vi "write_markerdata.vi"(0 "Data to save in":dbl[][](array[numeric]), 1 "Connected to Unity last call? In":bool, 2 "Connected to Unity via TCP?":bool, 3 "Host folder":path=path "C:/Users/User/Documents/GitHub/RobUST/Labview/RobUST_3D/Recorded Data", 4 "Unity task info string":string, 5 "DesiredTensions":dbl[](array[numeric]), 6 "Current save file in":path, 7 "CurrentTensions":dbl[](array[numeric]), 8 "New task info string flag in":bool, 9 "Last Vicon frame read":u32, 10 "Task has ended flag":bool) -> (14 "Connected to Unity last call? Out":bool, 15 "Current save file out":path, 16 "Data to save":dbl[][](array[numeric]), 17 "New task info string flag out":bool, 18 "Task had ended flag out":bool)   [LabVIEW 2024]
panel:
  in  "Actively record tensions":bool
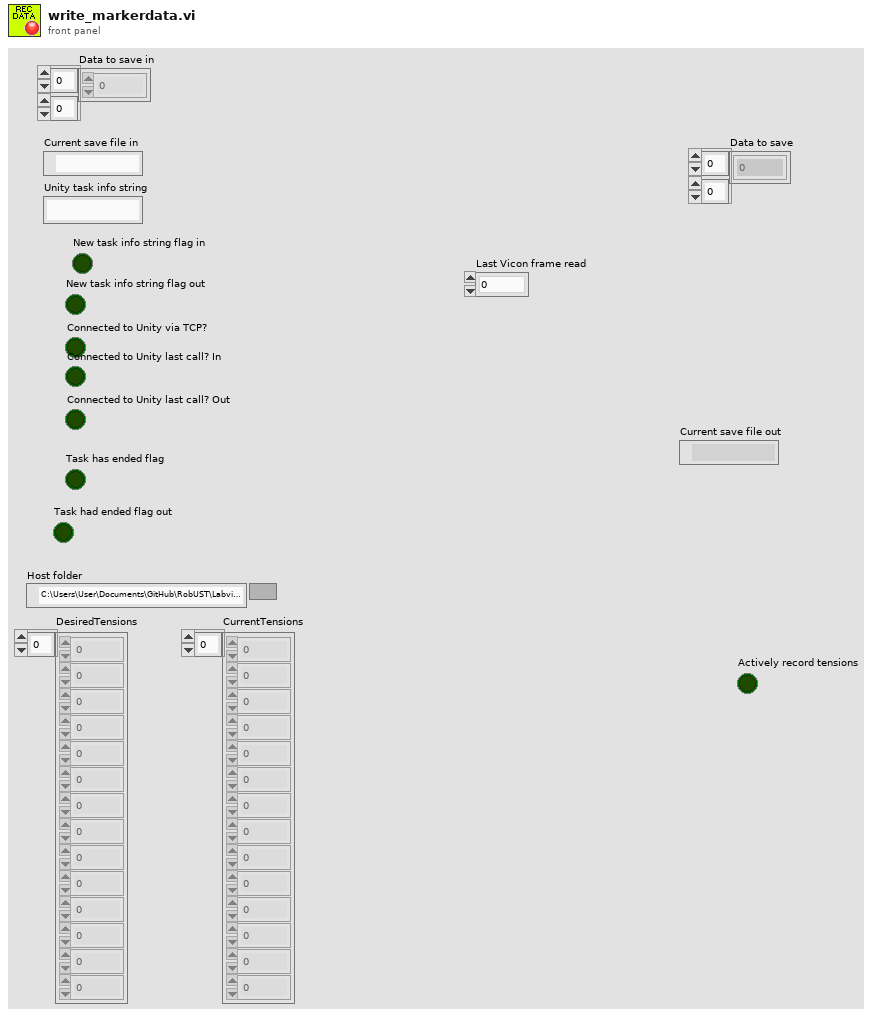
[diagram p1: front panel]
types:
  T1 = enum16{"open", "replace", "create", "open or create", "replace or create", "replace or create with confirmation"}
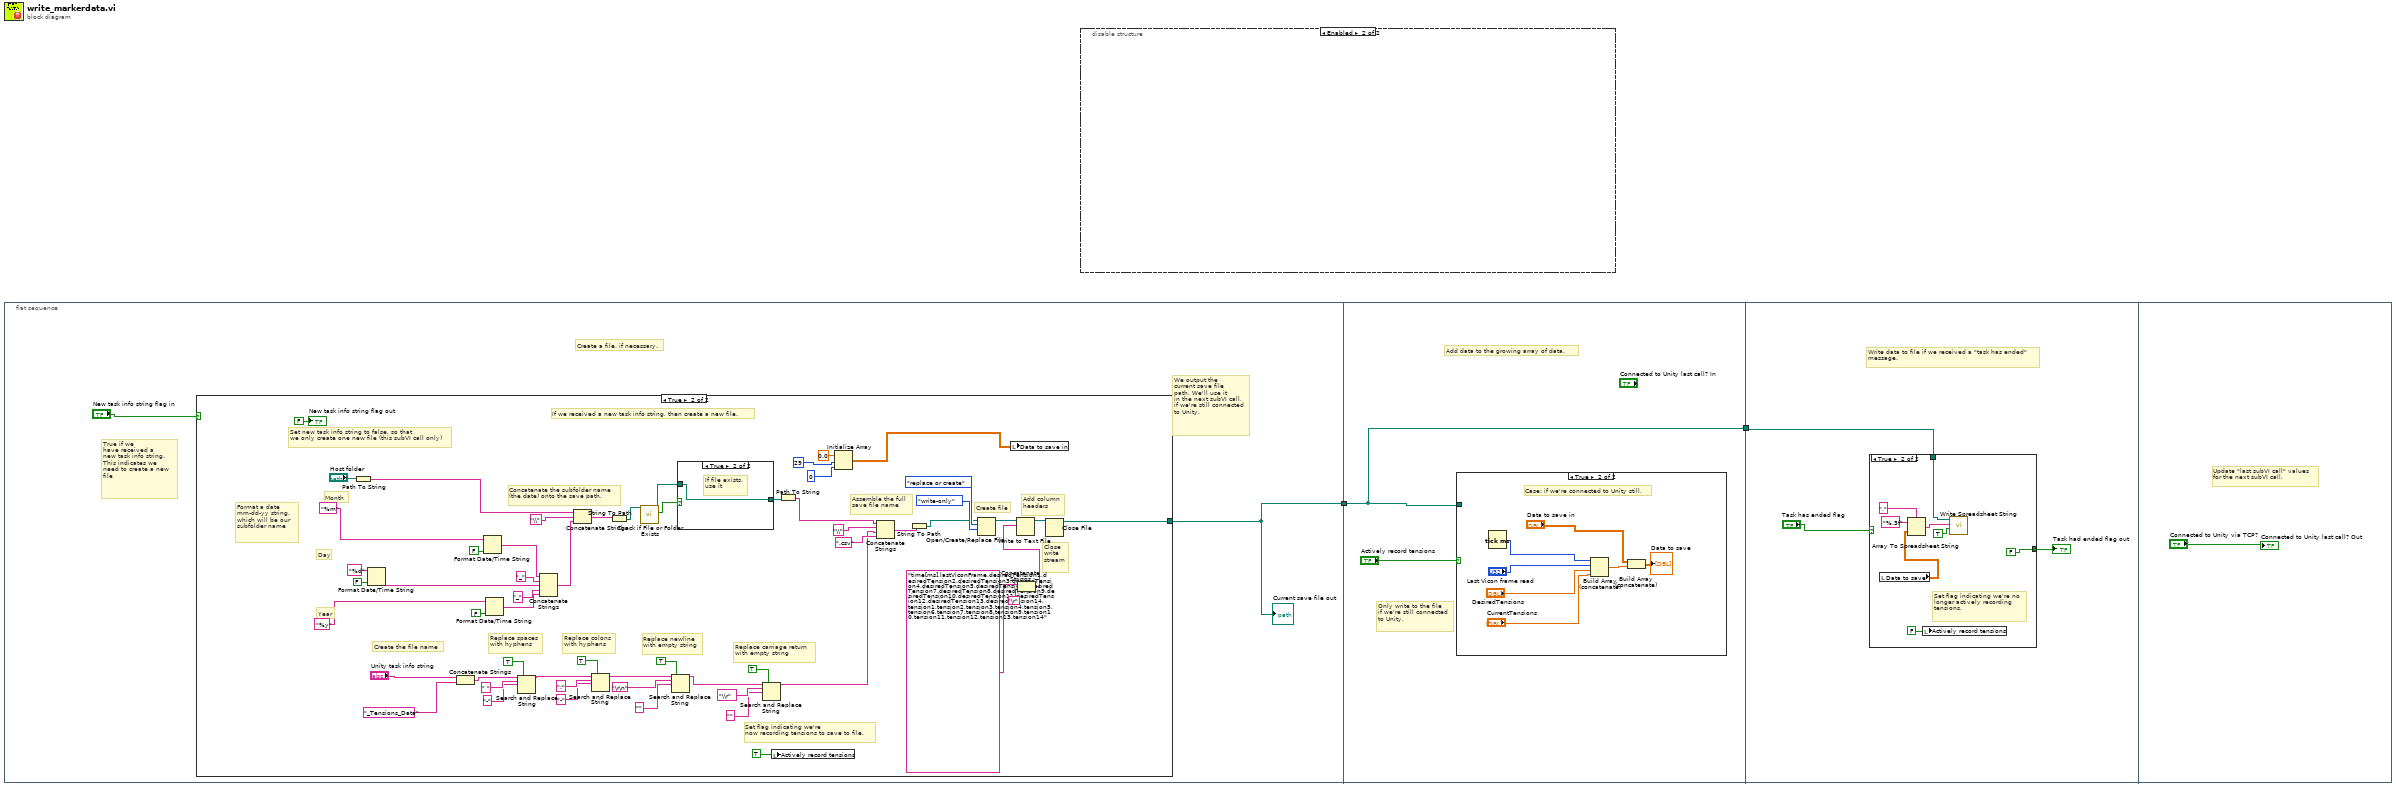
[diagram p0: block diagram]
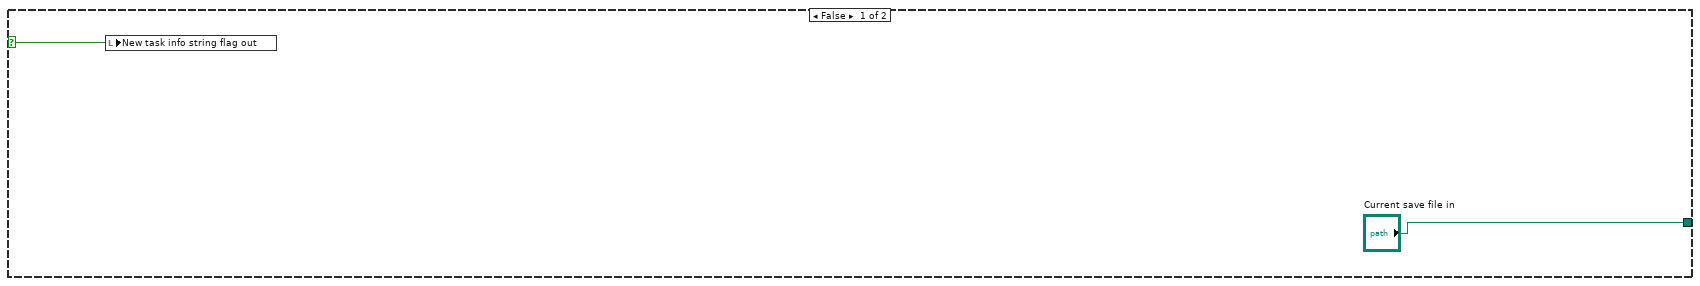
[diagram p2: hidden frame]
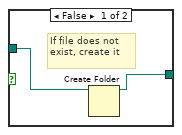
[diagram p3: hidden frame]
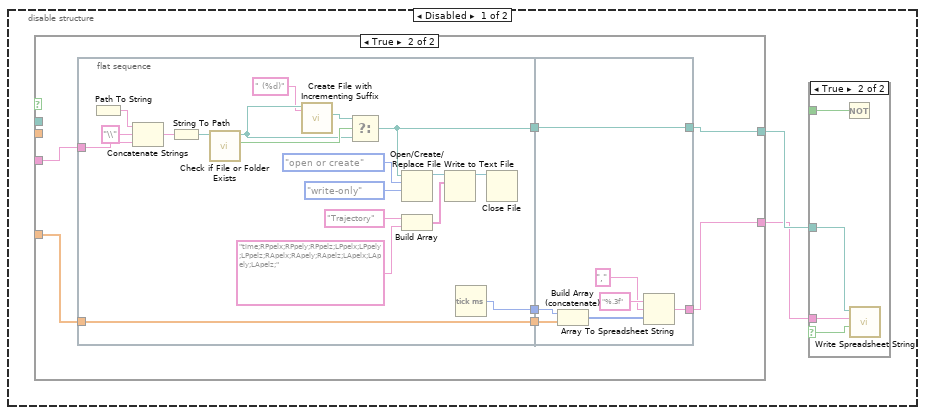
[diagram p6: hidden frame]
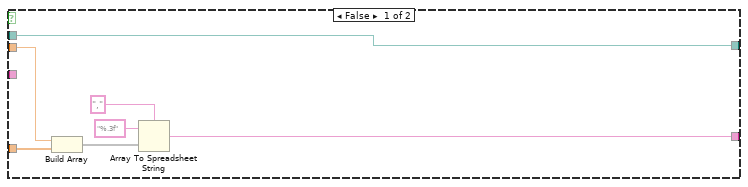
[diagram p7: hidden frame]
diagram:
  n1 = flat-sequence {
    tunnel: [w4] -> w2
    tunnel: w2 -> [w69]
    tunnel: [w69] -> w1
    tunnel: w1 -> [w79]
    frame #0 {
      # "We output the \ncurrent save file\npath. We'll use it \nin the next subVI call,\nif we're still connected\nto Unity."
      # "True if we \nhave received a \nnew task info string. \nThis indicates we \nneed to create a new \nfile"
      # "Create a file, if necessary."
      n2 = case shown="True" "New task info string flag in" {
        selector: "New task info string flag in" -> [w5 _]
        tunnel: ["Current save file in" w41] -> w4
        frame False {
          n3 = local write "New task info string flag out"(w5) -> ()
        }
        frame True {
          # "Day"
          # "Replace carriage return\nwith empty string"
          # "Replace newline\nwith empty string"
          # "Set flag indicating we're \nnow recording tensions to save to file."
          # "Set new task info string to false, so that\nwe only create one new file (this subVI call only)"
          # "Replace colons\nwith hyphens"
          # "Replace spaces\nwith hyphens"
          # "Close \nwrite\nstream"
          # "Add column\nheaders"
          # "Create file"
          # "Assemble the full \nsave file name"
          # "Create the file name"
          # "If we received a new task info string, then create a new file."
          # "Concatenate the subfolder name\n(the date) onto the save path."
          # "Format a date\nmm-dd-yy string, \nwhich will be our \nsubfolder name"
          # "Year"
          # "Month"
          n4 = Path To String(path="Host folder") -> (string=w63:string)
          n5 = Format Date/Time String(time format string (%c)="%d", UTC format=FALSE) -> (date/time string=w8:string)  [unwired: 1 in]
          n6 = Concatenate Strings("Unity task info string", "_Tensions_Data" ("string")) -> (w40:string)
          n7 = Format Date/Time String(time format string (%c)="%m", UTC format=FALSE) -> (date/time string=w62:string)  [unwired: 1 in]
          n8 = Format Date/Time String(time format string (%c)="%y", UTC format=FALSE) -> (date/time string=w9:string)  [unwired: 1 in]
          n9 = Search and Replace String(replace all?=TRUE ("replace all? (F)"), input string=w40, search string=" ", replace string="-" ("replace string (\"\")")) -> (result string=w33:string)  [unwired: 4 in, 3 out]
          n10 = Concatenate Strings(w62, "_" ("string"), w8, "_" ("string"), w9) -> (w64:string)
          n11 = Concatenate Strings(w63, "\\" ("string"), w64) -> (w49:string)
          n12 = Search and Replace String(replace all?=TRUE ("replace all? (F)"), input string=w33, search string=":", replace string="-" ("replace string (\"\")")) -> (result string=w18:string)  [unwired: 4 in, 3 out]
          n13 = String To Path(string=w49) -> (path=w52:path)
          n14 = call <vilib>:"Check if File or Folder Exists.vi"("path"=w52) -> ("file or folder exists?"=w51:bool, "dup path"=w50:path)  [unwired: 8 in, 1 out]
          n15 = Search and Replace String(replace all?=TRUE ("replace all? (F)"), input string=w18, search string="\r\n", replace string="" ("replace string (\"\")")) -> (result string=w14:string)  [unwired: 4 in, 3 out]
          n16 = case shown="True" w51 {
            tunnel: w50 -> [w66 w67]
            tunnel: [w65 w67] -> w48
            frame False {
              # "If file does not\nexist, create it"
              n17 = Create Folder(path (use dialog)=w66) -> (created path=w65:path)  [unwired: 2 in, 2 out]
            }
            frame True {
              # "If file exists, \nuse it"
            }
          }
          n18 = Search and Replace String(replace all?=TRUE ("replace all? (F)"), input string=w14, search string="\\r", replace string="" ("replace string (\"\")")) -> (result string=w13:string)  [unwired: 4 in, 3 out]
          n19 = local write "Actively record tensions"(TRUE ("Actively record tensions")) -> ()
          n20 = Path To String(path=w48) -> (string=w47:string)
          n21 = Initialize Array(0.0 ("element"), 29 ("dimension size"), 0 ("dimension size")) -> (w30:dbl[][])
          n22 = Concatenate Strings(w47, "\\" ("string"), w13, ".csv" ("string")) -> (w53:string)
          n23 = String To Path(string=w53) -> (path=w43:path)
          n24 = Open/Create/Replace File(file path (use dialog)=w43, operation (0:open)=T1."replace or create", access (0:read/write)=enum16{"read/write", "read-only", "write-only"}."write-only") -> (refnum out=w44:refnum<file>)  [unwired: 3 in, 2 out]
          n25 = local write "Data to save in"(w30) -> ()
          n26 = Concatenate Strings("time[ms],lastViconFrame,desiredTension1,desiredTension2,desiredTension3,desiredTension4,desiredTension5,desiredTension6,desiredTension7,desiredTension8,desiredTension9,desiredTension10,desiredTension11,desiredTension12,desiredTension13,desiredTension14, tension1,tension2,tension3,tension4,tension5,tension6,tension7,tension8,tension9,tension10,tension11,tension12,tension13,tension14" ("String"), "\r") -> (w27:string)
          n27 = Write to Text File(file (use dialog)=w44, text=w27) -> (refnum out=w42:refnum<file>)  [unwired: 2 in, 2 out]
          n28 = Close File(refnum=w42) -> (path=w41:path)  [unwired: 1 in, 1 out]
          "New task info string flag out" <- FALSE ("New task info string flag out")
        }
      }
      "Current save file out" <- w4
    }
    frame #1 {
      # "Add data to the growing array of data."
      # "Only write to the file\nif we're still connected\nto Unity."
      n29 = case shown="True" "Actively record tensions" {
        tunnel: w69 -> [_ _]
        frame False {
          # "If we're not currently connected \nto Unity, do nothing."
        }
        frame True {
          # "Case: if we're connected to Unity still."
          n30 = Tick Count (ms)() -> (millisecond timer value=w76:u32)
          n31 = Build Array (concatenate)(w76, "Last Vicon frame read", "DesiredTensions", "CurrentTensions") -> (w75:dbl[])
          n32 = Build Array (concatenate)("Data to save in", w75) -> (→"Data to save":dbl[][])
        }
      }
    }
    frame #2 {
      # "Write data to file if we received a \"task has ended\"\nmessage."
      n33 = case shown="True" "Task has ended flag" {
        selector: "Task has ended flag" -> [w80 _]
        tunnel: w79 -> [_ w84]
        tunnel: [w80 FALSE ("Task had ended flag out")] -> w77
        frame False {
        }
        frame True {
          # "Set flag indicating we're no\nlonger actively recording \ntensions."
          n34 = local read "Data to save"() -> (w83:dbl[][])
          n35 = Array To Spreadsheet String(delimiter (Tab)="," ("delimiter (\\t)"), array=w83, 3:"%.3f" ("format string")) -> (spreadsheet string=w88:string)
          n36 = local write "Actively record tensions"(FALSE ("Actively record tensions")) -> ()
          n37 = call <vilib>:"Write Spreadsheet String.vi"("append to file? (new file:F)"=TRUE, "spreadsheet string"=w88, "file path (dialog if empty)"=w84) -> ()  [unwired: 7 in, 2 out]
        }
      }
      "Task had ended flag out" <- w77
    }
    frame #3 {
      # "Update \"last subVI call\" values \nfor the next subVI call."
      "Connected to Unity last call? Out" <- "Connected to Unity via TCP?"
    }
  }
  n38 = disable-structure shown="Enabled" {
    frame Disabled {
      n39 = case shown="True" {
        selector: _ -> [_ _]
        tunnel: [w98 w104] -> w91
        tunnel: _ -> [w98 _]
        tunnel: _ -> [_ w105]
        tunnel: _ -> [w96 w100]
        tunnel: _ -> [w97 _]
        tunnel: [w94 w99] -> w90
        frame False {
          n40 = Build Array(w97, w96) -> (w95:void[])
          n41 = Array To Spreadsheet String(delimiter (Tab)="," ("delimiter (\\t)"), array=w95, 3:"%.3f" ("format string")) -> (spreadsheet string=w94:string)
        }
        frame True {
          n42 = flat-sequence {
            tunnel: w105 -> [w109]
            tunnel: [w113] -> w103
            tunnel: [w106] -> w102
            tunnel: [w111] -> w101
            tunnel: w100 -> [w111]
            tunnel: [w131] -> w104
            tunnel: w103 -> [w131]
            tunnel: w102 -> [w127]
            tunnel: w101 -> [w126]
            tunnel: [w125] -> w99
            frame #0 {
              n43 = Path To String() -> (string=w121:string)  [unwired: 1 in]
              n44 = Concatenate Strings(w121, "\\" ("string"), w109) -> (w120:string)
              n45 = String To Path(string=w120) -> (path=w123:path)
              n46 = call <vilib>:"Check if File or Folder Exists.vi"("path"=w123) -> ("file or folder exists?"=w124:bool, "dup path"=w119:path)  [unwired: 8 in, 1 out]
              n47 = call <vilib>:"Create File with Incrementing Suffix.vi"("format string (\" (%d)\")"=" (%d)" ("format string (\" (%d)\")"), "file path"=w119) -> ("actual path"=w118:path)  [unwired: 7 in, 2 out]
              n48 = Select(t=w118, s=w124, f=w119) -> (s? t:f=w113:path)
              n49 = Open/Create/Replace File(file path (use dialog)=w113, operation (0:open)=T1."open or create", access (0:read/write)=enum16{"read/write", "read-only", "write-only"}."write-only") -> (refnum out=w114:refnum<file>)  [unwired: 3 in, 2 out]
              n50 = Build Array("Trajectory" ("element"), "time;RPpelx;RPpely;RPpelz;LPpelx;LPpely;LPpelz;RApelx;RApely;RApelz;LApelx;LApely;LApelz;" ("String")) -> (w110:string[])
              n51 = Write to Text File(file (use dialog)=w114, text=w110) -> (refnum out=w112:refnum<file>)  [unwired: 2 in, 2 out]
              n52 = Tick Count (ms)() -> (millisecond timer value=w106:u32)
              n53 = Close File(refnum=w112) -> ()  [unwired: 1 in, 2 out]
            }
            frame #1 {
              n54 = Build Array (concatenate)(w127, w126) -> (w130:u32[])
              n55 = Array To Spreadsheet String(delimiter (Tab)="," ("delimiter (\\t)"), array=w130, 3:"%.3f" ("format string")) -> (spreadsheet string=w125:string)
            }
          }
        }
      }
      n56 = case shown="True" {
        selector: _ -> [_ w132]
        tunnel: w91 -> [_ w135]
        tunnel: _ -> [_ w133]
        tunnel: w90 -> [_ w134]
        frame False {
        }
        frame True {
          n57 = Not(x=w133) -> ()  [unwired: 1 out]
          n58 = call <vilib>:"Write Spreadsheet String.vi"("append to file? (new file:F)"=w132, "spreadsheet string"=w134, "file path (dialog if empty)"=w135) -> ()  [unwired: 7 in, 2 out]
        }
      }
    }
    frame Enabled {
    }
  }
